vi "Var-Name-Manipulator-for-ODE-plots.vi"(8 "error in (no error)":errorcluster, 9 "In_ODE":string[](array[string])=["-(kd*CI)+10*((ko__P1*ng__P1*Ko__P1*RNAP)/(1+Ko__P1*RNAP+(Kr__LacI_P1*LacI)^nc__LacI_P1))+10*((ko__P2*ng__P2*Ko__P2*RNAP)/(1+Ko__P2*RNAP+(Kr__TetR_P2*TetR)^nc__TetR_P2))", "-(kd*GFP)+10*((ko__Promoter_GFP*ng__Promoter_GFP*Ko__Promoter_GFP*RNAP)/(1+Ko__Promoter_GFP*RNAP+(Kr__CI_Promoter_GFP*CI)^nc__CI_Promoter_GFP))"], 10 "In_Tot_Param":string[](array[string])=["ko_r", "nr", "np", "kr_r", "ka_f", "kecdiff", "ko", "kmdiff_f", "kecd", "kc_r", "kr_f", "ka_r", "nc", "kao_r", "kd", "kb", "ng", "ka", "kao_f", "kmdiff_r", "ko_f", "kc_f", "High", "HighTime", "HighTime2", "kd", "kd", "kd", "kd", "RNAP", "ng__P1", "Ko__P1", "ko__P1", "nc__LacI_P1", "Kr__LacI_P1", "RNAP", "ng__P2", "Ko__P2", "ko__P2", "nc__TetR_P2", "Kr__TetR_P2", "RNAP", "ng__Promoter_GFP", "Ko__Promoter_GFP", "ko__Promoter_GFP", "nc__CI_Promoter_GFP", "Kr__CI_Promoter_GFP"], 11 "In_X_for_ODE":string[](array[string])=["CI", "GFP"]) -> (0 "error out":errorcluster, 1 "Out_ODE":string[](array[string]), 2 "Out_Tot_Param":string[](array[string]), 3 "Out_X_for_ODE":string[](array[string]))   [LabVIEW 2014]
doc: "This VI manipulates the variable and parameters name according to the format acceptable to LabVIEW ODE VI.\n\nDesigned By: HB\nhaba@dtu.dk"
uses:
  <vilib>/regexp/Match Regular Expression.xnode
panel:
  out "offset past match":i32
  out "L-Op":string
  out "R-Op":string
  out "ODE":string[][](table)
  out "Parameters":string[][](table)
  out "X Variables":string[][](table)
  out "Cnt_digit":i32
  out "Cnt_Char":i32
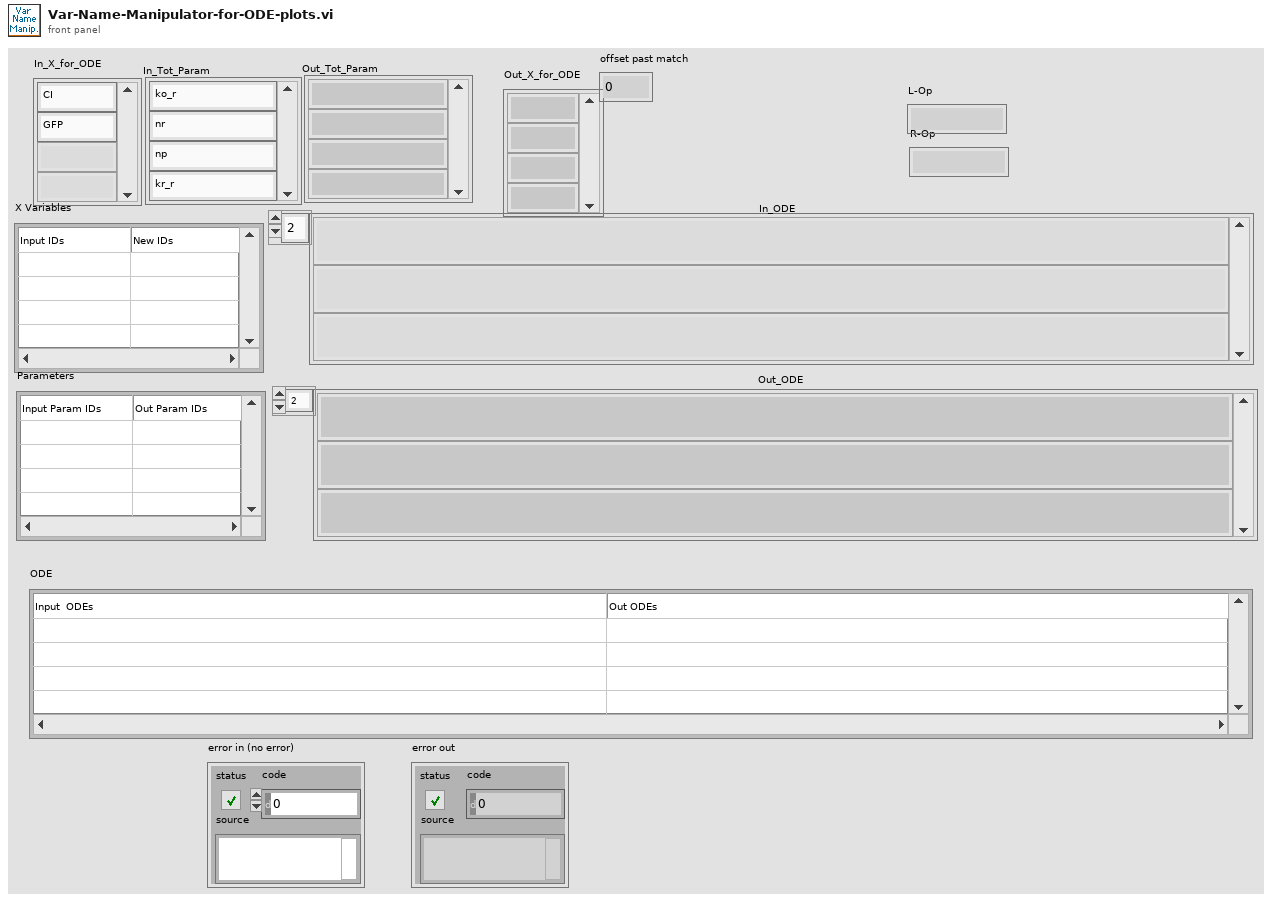
[diagram p1: front panel]
types:
  T1 = enum16{"big-endian, network order", "native, host order", "little-endian"}
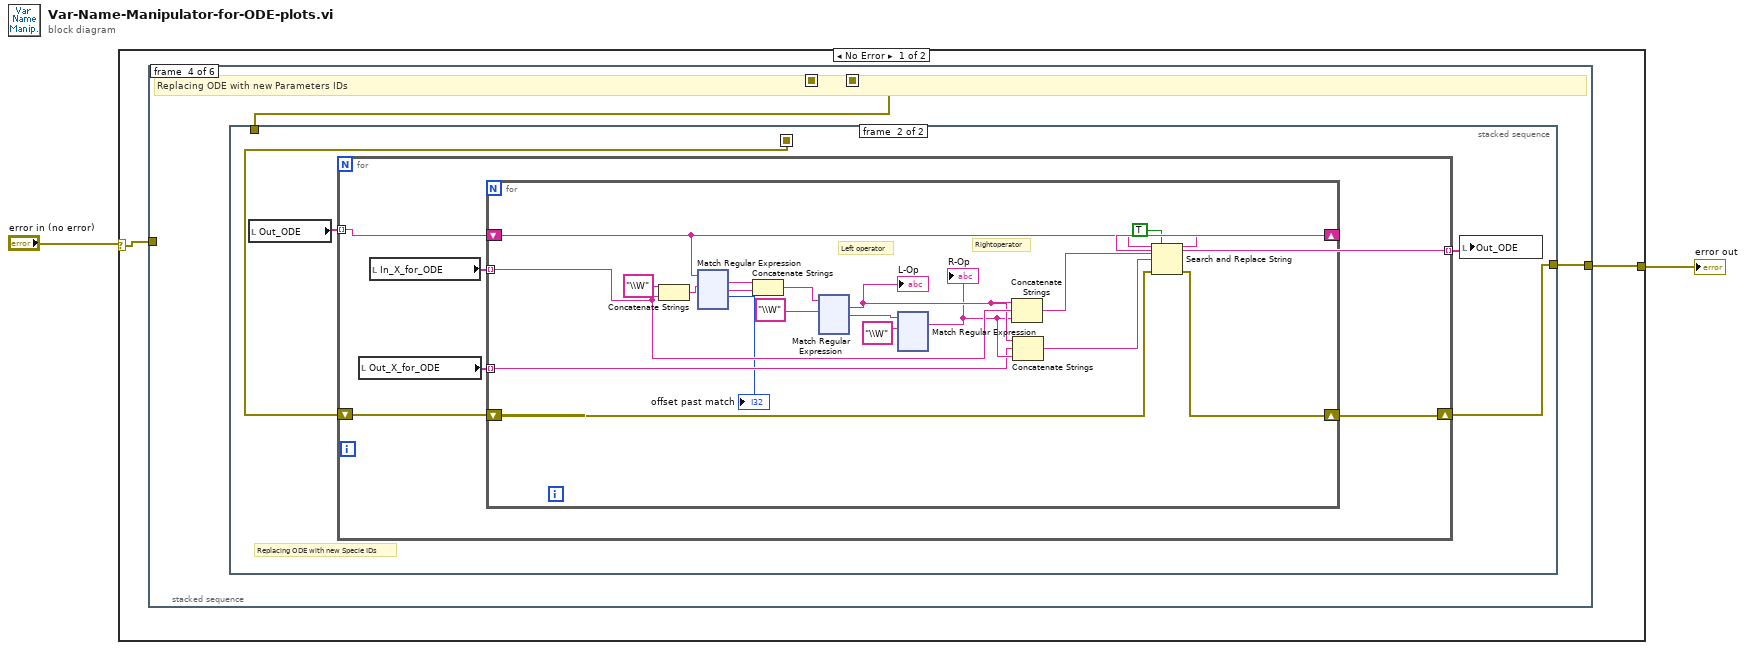
[diagram p0: block diagram]
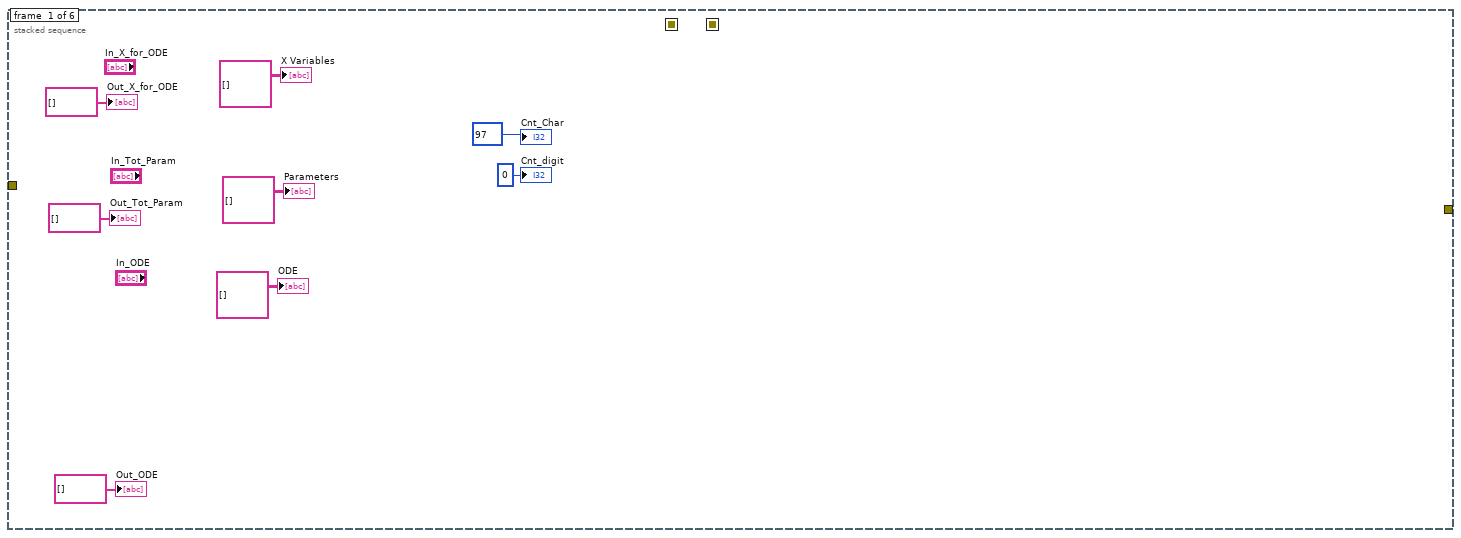
[diagram p2: hidden frame]
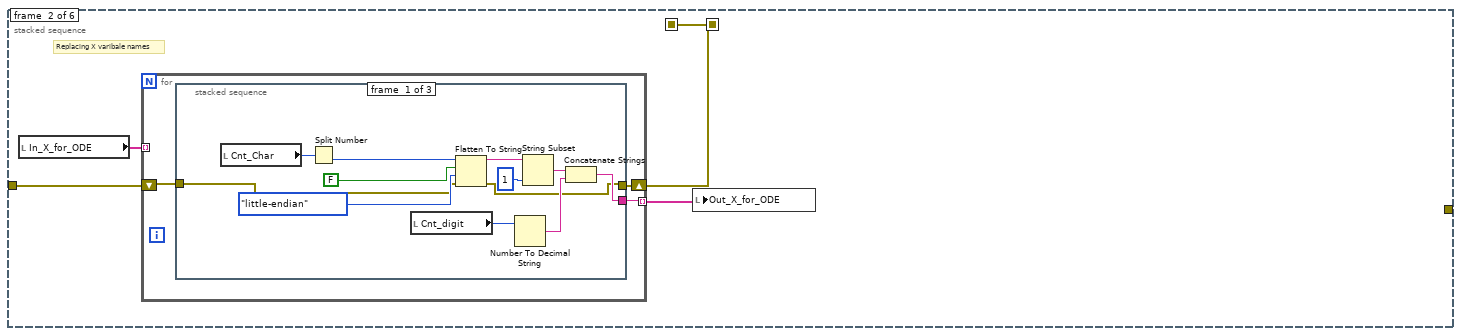
[diagram p3: hidden frame]
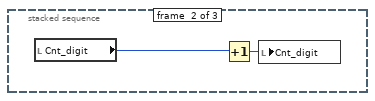
[diagram p4: hidden frame]
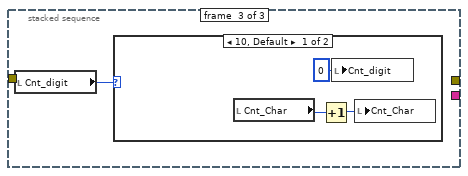
[diagram p5: hidden frame]
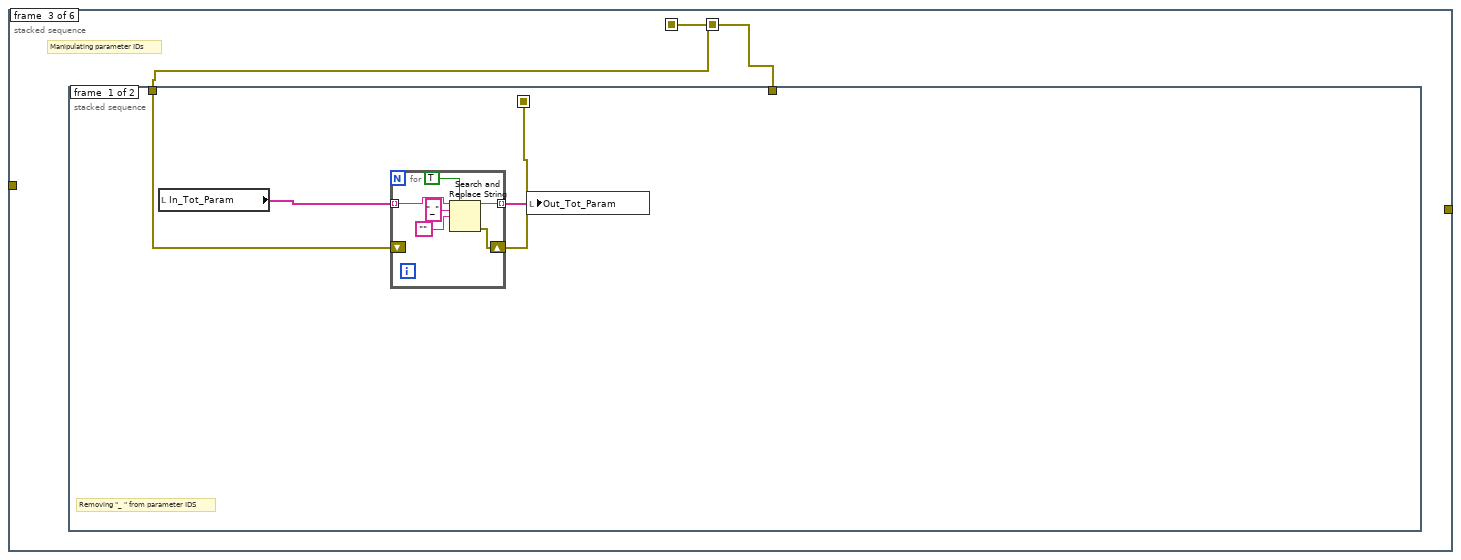
[diagram p7: hidden frame]
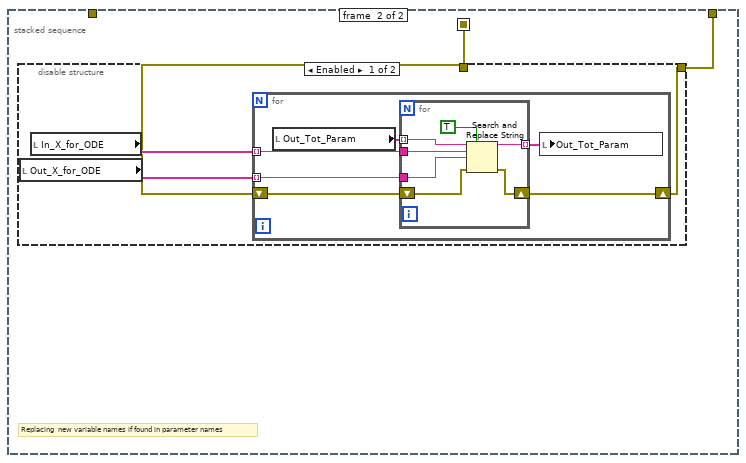
[diagram p8: hidden frame]
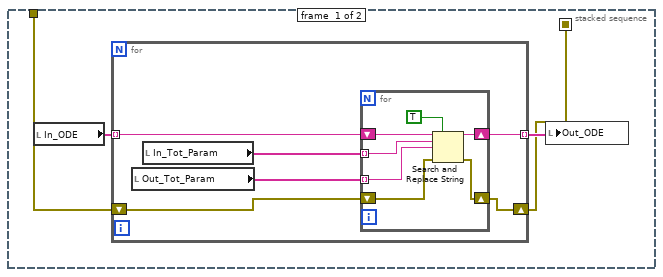
[diagram p10: hidden frame]
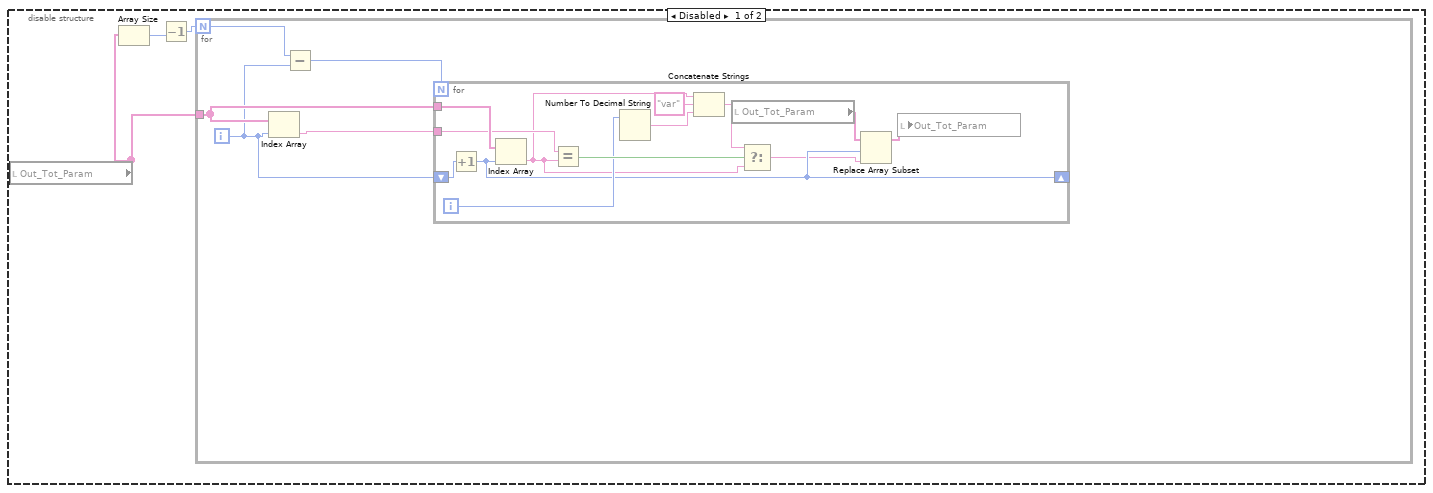
[diagram p12: hidden frame]
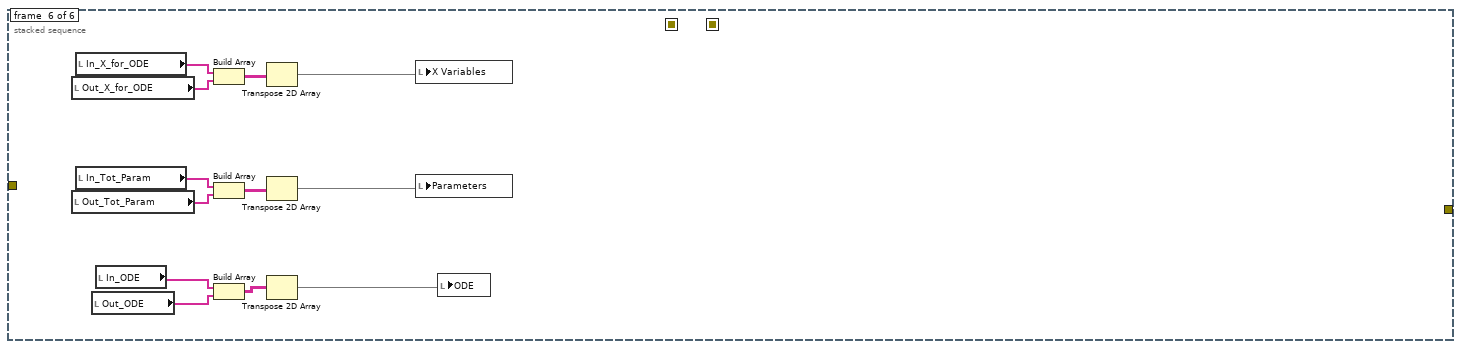
[diagram p13: hidden frame]
diagram:
  n1 = case shown="No Error" "error in (no error)" {
    selector: "error in (no error)" -> [w4 w494]
    tunnel: [w3 w494] -> w1
    frame No Error {
      n2 = stacked-sequence {
        seq-local: [_ w13 _ _ _ _] -> [_ _ w39 _ _ _]
        seq-local: [_ _ w38 _ _ _] -> [_ _ _ w71 _ _]
        tunnel: w4 -> [_ w14 _ _ _ _]
        tunnel: [_ _ _ w70 _ _] -> w3
        frame #0 {
          "Out_X_for_ODE" <- string[] [] ("X_Replaced_with")
          "Cnt_Char" <- 97
          "Cnt_digit" <- 0 ("Cnt_digit")
          "Out_Tot_Param" <- string[] [] ("Param_Replaced_with")
          "Out_ODE" <- string[] [] ("Out_ODe")
          "X Variables" <- string[][] [] ("X Variables")
          "Parameters" <- string[][] [] ("X Variables")
          "ODE" <- string[][] [] ("X Variables")
        }
        frame #1 {
          # "Replacing X varibale names"
          n3 = local read "In_X_for_ODE"() -> (w16:string[])
          n4 = for {
            tunnel: w16 -> [_] mode=indexing
            tunnel: [w19] -> w15 mode=indexing
            shift-right: [w17] -> w13
            shift-left: w14 -> [w18]
            n5 = stacked-sequence {
              tunnel: [w22 _ _] -> w19
              tunnel: w18 -> [w21 _ _]
              tunnel: [w20 _ _] -> w17
              frame #0 {
                n6 = local read "Cnt_Char"() -> (w28:i32)
                n7 = Split Number(x=w28) -> (lo(x)=w31:u16)  [unwired: 1 out]
                n8 = local read "Cnt_digit"() -> (w27:i32)
                n9 = Flatten To String(anything=w31, prepend array or string size? (T)=FALSE, byte order (0:big-endian, network order)=T1."little-endian", error in (no error)=w21) -> (data string=w25:string, error out=w20:errorcluster)  [unwired: 1 out]
                n10 = Number To Decimal String(number=w27) -> (decimal integer string=w23:string)  [unwired: 1 in]
                n11 = String Subset(string=w25, length (rest)=1 ("length (rest)")) -> (substring=w24:string)  [unwired: 1 in]
                n12 = Concatenate Strings(w24, w23) -> (w22:string)
              }
              frame #1 {
                n13 = local read "Cnt_digit"() -> (w33:i32)
                n14 = Increment(x=w33) -> (x+1=w32:i32)
                n15 = local write "Cnt_digit"(w32) -> ()
              }
              frame #2 {
                n16 = local read "Cnt_digit"() -> (w34:i32)
                n17 = case shown="10, Default" w34 {
                  frame 10, Default {
                    n18 = local read "Cnt_Char"() -> (w36:i32)
                    n19 = Increment(x=w36) -> (x+1=w35:i32)
                    n20 = local write "Cnt_digit"(0 ("Cnt_digit")) -> ()
                    n21 = local write "Cnt_Char"(w35) -> ()
                  }
                  frame 0..9 {
                  }
                }
              }
            }
          }
          n22 = local write "Out_X_for_ODE"(w15) -> ()
        }
        frame #2 {
          # "Manipulating parameter IDs"
          n23 = stacked-sequence {
            seq-local: [w40 _] -> [_ w51]
            tunnel: w39 -> [w41 _]
            tunnel: [_ w50] -> w38
            frame #0 {
              # "Removing \"_ \" from parameter IDS"
              n24 = local read "In_Tot_Param"() -> (w43:string[])
              n25 = for {
                tunnel: w43 -> [w49] mode=indexing
                tunnel: [w46] -> w42 mode=indexing
                shift-right: [w44] -> w40
                shift-left: w41 -> [_]
                n26 = Search and Replace String(replace all?=TRUE ("replace all? (F)"), input string=w49, search string="_", replace string="") -> (result string=w46:string, error out=w44:errorcluster)  [unwired: 4 in, 2 out]
              }
              n27 = local write "Out_Tot_Param"(w42) -> ()
            }
            frame #1 {
              # "Replacing  new variable names if found in parameter names"
              n28 = disable-structure shown="Enabled" {
                disable-tunnel: w51 -> [w53 w69]
                disable-tunnel: [w52 w69] -> w50
                frame Enabled {
                  n29 = local read "Out_X_for_ODE"() -> (w54:string[])
                  n30 = local read "In_X_for_ODE"() -> (w55:string[])
                  n31 = for {
                    tunnel: w55 -> [w58] mode=indexing
                    tunnel: w54 -> [w60] mode=indexing
                    shift-right: [w57] -> w52
                    shift-left: w53 -> [w56]
                    n32 = local read "Out_Tot_Param"() -> (w61:string[])
                    n33 = for {
                      tunnel: w61 -> [w65] mode=indexing
                      tunnel: w60 -> [w68]
                      tunnel: [w66] -> w59 mode=indexing
                      tunnel: w58 -> [w64]
                      shift-right: [w63] -> w57
                      shift-left: w56 -> [w62]
                      n34 = Search and Replace String(replace all?=TRUE ("replace all? (F)"), input string=w65, search string=w64, replace string=w68, error in=w62) -> (result string=w66:string, error out=w63:errorcluster)  [unwired: 3 in, 2 out]
                    }
                    n35 = local write "Out_Tot_Param"(w59) -> ()
                  }
                }
                frame Disabled {
                }
              }
            }
          }
        }
        frame #3 {
          # "Replacing ODE with new Parameters IDs"
          n36 = stacked-sequence {
            seq-local: [w72 _] -> [_ w90]
            tunnel: w71 -> [w73 _]
            tunnel: [_ w89] -> w70
            frame #0 {
              n37 = local read "In_ODE"() -> (w75:string[])
              n38 = for {
                tunnel: w75 -> [w81] mode=indexing
                tunnel: [w78] -> w74 mode=indexing
                shift-right: [w77] -> w72
                shift-left: w73 -> [w76]
                n39 = local read "Out_Tot_Param"() -> (w79:string[])
                n40 = local read "In_Tot_Param"() -> (w80:string[])
                n41 = for {
                  tunnel: w80 -> [w87] mode=indexing
                  tunnel: w79 -> [w86] mode=indexing
                  shift-right: [w84] -> w78
                  shift-left: w81 -> [w88]
                  shift-right: [w83] -> w77
                  shift-left: w76 -> [w82]
                  n42 = Search and Replace String(replace all?=TRUE ("replace all? (F)"), input string=w88, search string=w87, replace string=w86, error in=w82) -> (result string=w84:string, error out=w83:errorcluster)  [unwired: 3 in, 2 out]
                }
              }
              n43 = local write "Out_ODE"(w74) -> ()
            }
            frame #1 {
              # "Replacing ODE with new Specie IDs"
              n44 = local read "Out_ODE"() -> (w92:string[])
              n45 = for {
                tunnel: w92 -> [w98] mode=indexing
                tunnel: [w95] -> w91 mode=indexing
                shift-right: [w94] -> w89
                shift-left: w90 -> [w93]
                n46 = local read "Out_X_for_ODE"() -> (w96:string[])
                n47 = local read "In_X_for_ODE"() -> (w97:string[])
                n48 = for {
                  tunnel: w97 -> [w105] mode=indexing
                  tunnel: w96 -> [w101] mode=indexing
                  shift-right: [w117] -> w95
                  shift-left: w98 -> [w106]
                  shift-right: [w115] -> w94
                  shift-left: w93 -> [w116]
                  # "Rightoperator"
                  # "Left operator"
                  n49 = Concatenate Strings("\\W" ("regular expression"), w105) -> (w112:string)
                  n50 = xnode "Match Regular Expression"("input string"=w106, "regular expression"=w112) -> ("whole match"=w111:string, "after match"=w110:string, "offset past match"=→"offset past match":i32)  [unwired: 4 in, 2 out]
                  n51 = Concatenate Strings(w111, w110) -> (w108:string)
                  n52 = xnode "Match Regular Expression"("input string"=w108, "regular expression"="\\W") -> ("whole match"=w103:string, "after match"=w107:string)  [unwired: 4 in, 3 out]
                  "L-Op" <- w103
                  n53 = xnode "Match Regular Expression"("input string"=w107, "regular expression"="\\W") -> ("whole match"=w102:string)  [unwired: 4 in, 4 out]
                  "R-Op" <- w102
                  n54 = Concatenate Strings(w103, w105, w102) -> (w104:string)
                  n55 = Concatenate Strings(w103, w101, w102) -> (w100:string)
                  n56 = Search and Replace String(replace all?=TRUE ("replace all? (F)"), input string=w106, search string=w104, replace string=w100, error in=w116) -> (result string=w117:string, error out=w115:errorcluster)  [unwired: 3 in, 2 out]
                }
              }
              n57 = local write "Out_ODE"(w91) -> ()
            }
          }
        }
        frame #4 {
          n58 = disable-structure shown="Enabled" {
            frame Disabled {
              n59 = local read "Out_Tot_Param"() -> (w463:string[])
              n60 = Array Size(array=w463) -> (size(s)=w462:i32)
              n61 = Decrement(x=w462) -> (x-1=w461:i32)
              n62 = for {
                N: w461 -> [w468]
                tunnel: w463 -> [w466]
                i -> [w464]
                n63 = Index Array(array=w466, index=w464) -> (element=w465:string)
                n64 = Subtract(x=w468, y=w464) -> (x-y=w467:i32)
                n65 = for {
                  N: w467 -> [_]
                  tunnel: w466 -> [w481]
                  tunnel: w465 -> [w480]
                  shift-right: [w471] -> _
                  shift-left: w464 -> [w478]
                  i -> [w474]
                  n66 = Increment(x=w478) -> (x+1=w471:i32)
                  n67 = Index Array(array=w481, index=w471) -> (element=w473:string)
                  n68 = Equal?(x=w480, y=w473) -> (x = y?=w479:bool)
                  n69 = Number To Decimal String(number=w474) -> (decimal integer string=w475:string)  [unwired: 1 in]
                  n70 = Concatenate Strings(w473, "var" ("string"), w475) -> (w477:string)
                  n71 = local read "Out_Tot_Param"() -> (w472:string[])
                  n72 = Select(t=w477, s=w479, f=w473) -> (s? t:f=w470:string)
                  n73 = Replace Array Subset(array=w472, new element=w470, index=w471) -> (w469:string[])
                  n74 = local write "Out_Tot_Param"(w469) -> ()
                }
              }
            }
            frame Enabled {
            }
          }
        }
        frame #5 {
          n75 = local read "Out_X_for_ODE"() -> (w491:string[])
          n76 = local read "Out_Tot_Param"() -> (w488:string[])
          n77 = local read "In_X_for_ODE"() -> (w492:string[])
          n78 = local read "In_Tot_Param"() -> (w487:string[])
          n79 = local read "Out_ODE"() -> (w483:string[])
          n80 = local read "In_ODE"() -> (w484:string[])
          n81 = Build Array(w492, w491) -> (w493:string[][])
          n82 = Build Array(w487, w488) -> (w486:string[][])
          n83 = Build Array(w484, w483) -> (w485:string[][])
          n84 = Transpose 2D Array(2D array=w493) -> (transposed array=w490:string[][])
          n85 = Transpose 2D Array(2D array=w486) -> (transposed array=w489:string[][])
          n86 = Transpose 2D Array(2D array=w485) -> (transposed array=w482:string[][])
          n87 = local write "X Variables"(w490) -> ()
          n88 = local write "Parameters"(w489) -> ()
          n89 = local write "ODE"(w482) -> ()
        }
      }
    }
    frame Error {
    }
  }
  "error out" <- w1
